vi "E4440A_PSA_Sweep_Coupling.vi"(0 "VISA resource name":refnum<visa-resource-name>, 1 "Enable Auto Video BandWidth (T: Enable)":bool=TRUE, 2 "Manual Video BandWidth (3 MHz)":i32=3000000, 5 "Enable Auto Sweep Time (T: Enable)":bool=TRUE, 7 "Manual Sweep Time (265 ms)":dbl=0.265, 9 "Enable Auto Resolution BandWidth (T: Enable)":bool=TRUE, 11 "error in (no error)":errorcluster, 12 "Manual Resolution BandWidth (3 MHz)":i32=3000000, 13 "Enable Auto VBW/RBW Ratio (T: Enable)":bool=TRUE, 14 "Manual VBW/RBW Ratio (1)":dbl=1.0) -> (4 "VISA resource name out":refnum<visa-resource-name>, 15 "error out":errorcluster)   [LabVIEW 2015]
doc: "Configures the coupling and sweeping properties of the spectrum analyzer. Resolution bandwidth, video bandwidth, and sweep time can be coupled together by the instrument or set manually."
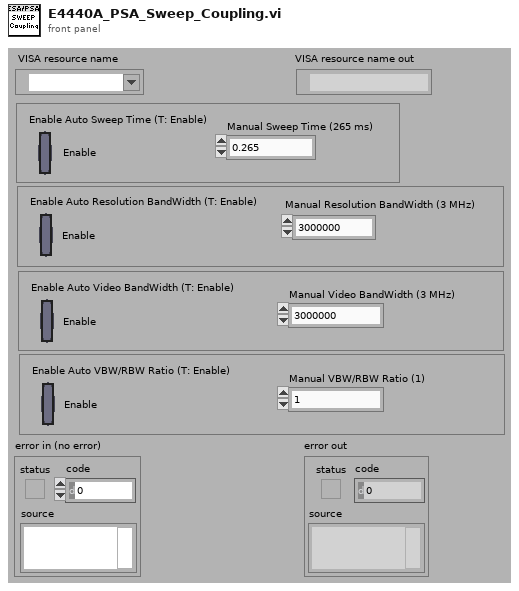
[diagram p1: front panel]
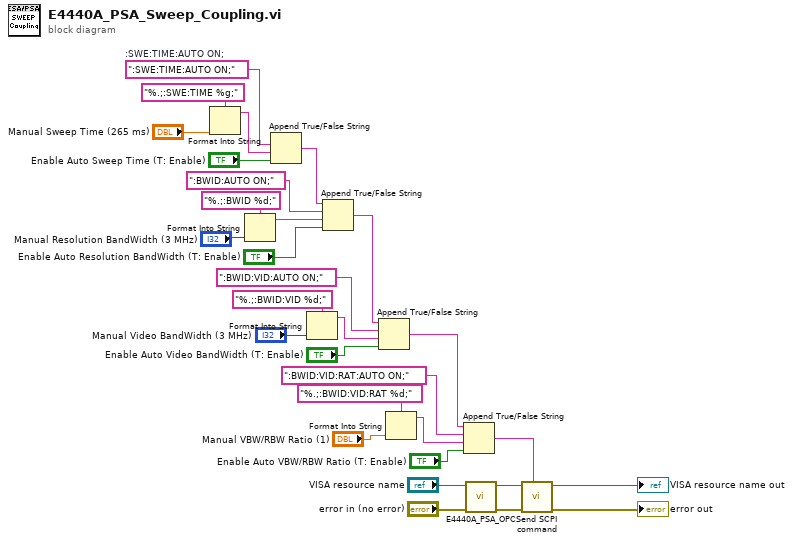
[diagram p0: block diagram]
diagram:
  w28 = ":SWE:TIME:AUTO ON;"  # :SWE:TIME:AUTO ON;
  n1 = Format Into String(format string="%.;:SWE:TIME %g;", "Manual Sweep Time (265 ms)") -> (resulting string=w27:string)  [unwired: 2 in, 1 out]
  n2 = Format Into String(format string="%.;:BWID %d;", "Manual Resolution BandWidth (3 MHz)") -> (resulting string=w20:string)  [unwired: 2 in, 1 out]
  n3 = Append True/False String(1:"Enable Auto Sweep Time (T: Enable)", 2:w27, 3:w28) -> (0:w23:string)  [unwired: 1 in]
  n4 = Format Into String(format string="%.;:BWID:VID %d;", "Manual Video BandWidth (3 MHz)") -> (resulting string=w17:string)  [unwired: 2 in, 1 out]
  n5 = Append True/False String(1:"Enable Auto Resolution BandWidth (T: Enable)", 2:w20, 3:":BWID:AUTO ON;" ("true string"), 4:w23) -> (0:w14:string)
  n6 = Append True/False String(1:"Enable Auto Video BandWidth (T: Enable)", 2:w17, 3:":BWID:VID:AUTO ON;" ("true string"), 4:w14) -> (0:w8:string)
  n7 = Format Into String(format string="%.;:BWID:VID:RAT %d;", "Manual VBW/RBW Ratio (1)") -> (resulting string=w11:string)  [unwired: 2 in, 1 out]
  n8 = Append True/False String(1:"Enable Auto VBW/RBW Ratio (T: Enable)", 2:w11, 3:":BWID:VID:RAT:AUTO ON;" ("true string"), 4:w8) -> (0:w4:string)
  n9 = call "E4440A_PSA_OPC.vi"("error in (no error)"="error in (no error)", "VISA resource name"="VISA resource name") -> ("error out"=w3:errorcluster, "VISA resource name out"=w1:refnum<visa-resource-name>)  [unwired: 8 in]
  n10 = call "Send SCPI command.vi"("Send SCPI Command"=w4, "error in (no error)"=w3, "VISA resource name"=w1) -> ("error out"=→"error out":errorcluster, "VISA resource name out"=→"VISA resource name out":refnum<visa-resource-name>)  [unwired: 7 in]
